vi "PicoReadPicoSingleBuffers.vi"(1 "enabled array":i16[](array[numeric]), 2 "Buffer and Transfer Settings":T3={"startIndex"=0, "Samples"=1000000, "Down Sample Ratio"=1, "Down-Sample Mode"=2147483648} {"Down-Sample Mode" items=["None"=2147483648, "Aggregate"=1, "Decimate"=2, "Average"=4]; "Down Sample Ratio" step=1; "Samples" format="%_6p"}, 3 "Variant":string, 5 "Data Pointers":T2, 9 "Buffer Number":i32=1, 11 "error in (no error)":errorcluster) -> (6 "MaxBuffers (Max or non-aggregated)":T1, 8 "Min Buffers":T1, 15 "error out":errorcluster)   [LabVIEW 2010]
doc: "Read data from a single Picodata buffer."
uses:
  PicoBuffers.ctl
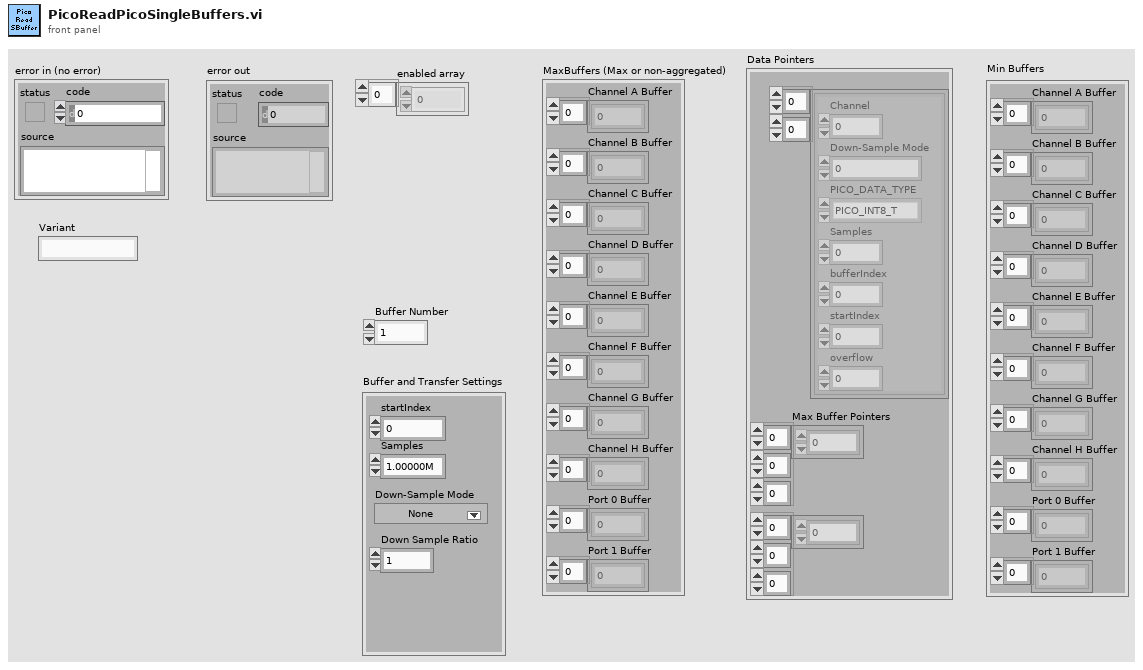
[diagram p1: front panel]
types:
  T1 = cluster{"Channel A Buffer":i16[], "Channel B Buffer":i16[], "Channel C Buffer":i16[], "Channel D Buffer":i16[], "Channel E Buffer":i16[], "Channel F Buffer":i16[], "Channel G Buffer":i16[], "Channel H Buffer":i16[], "Port 0 Buffer":i16[], "Port 1 Buffer":i16[]}
  T2 = typedef "PicoBuffers.ctl" = cluster{"Max Buffer Pointers":u64[][][], "Min Buffer Pointers":u64[][][], "StreamingDataInfo":cluster{"Channel":u32, "Down-Sample Mode":u32, "PICO_DATA_TYPE":enum32{"PICO_INT8_T", "PICO_INT16_T", "PICO_INT32_T", "PICO_UINT32_T", "PICO_INT64_T", ""}, "Samples":i32, "bufferIndex":u64, "startIndex":i32, "overflow":i16}[][]}
  T3 = cluster{"startIndex":u64, "Samples":u64, "Down Sample Ratio":u64, "Down-Sample Mode":u32}
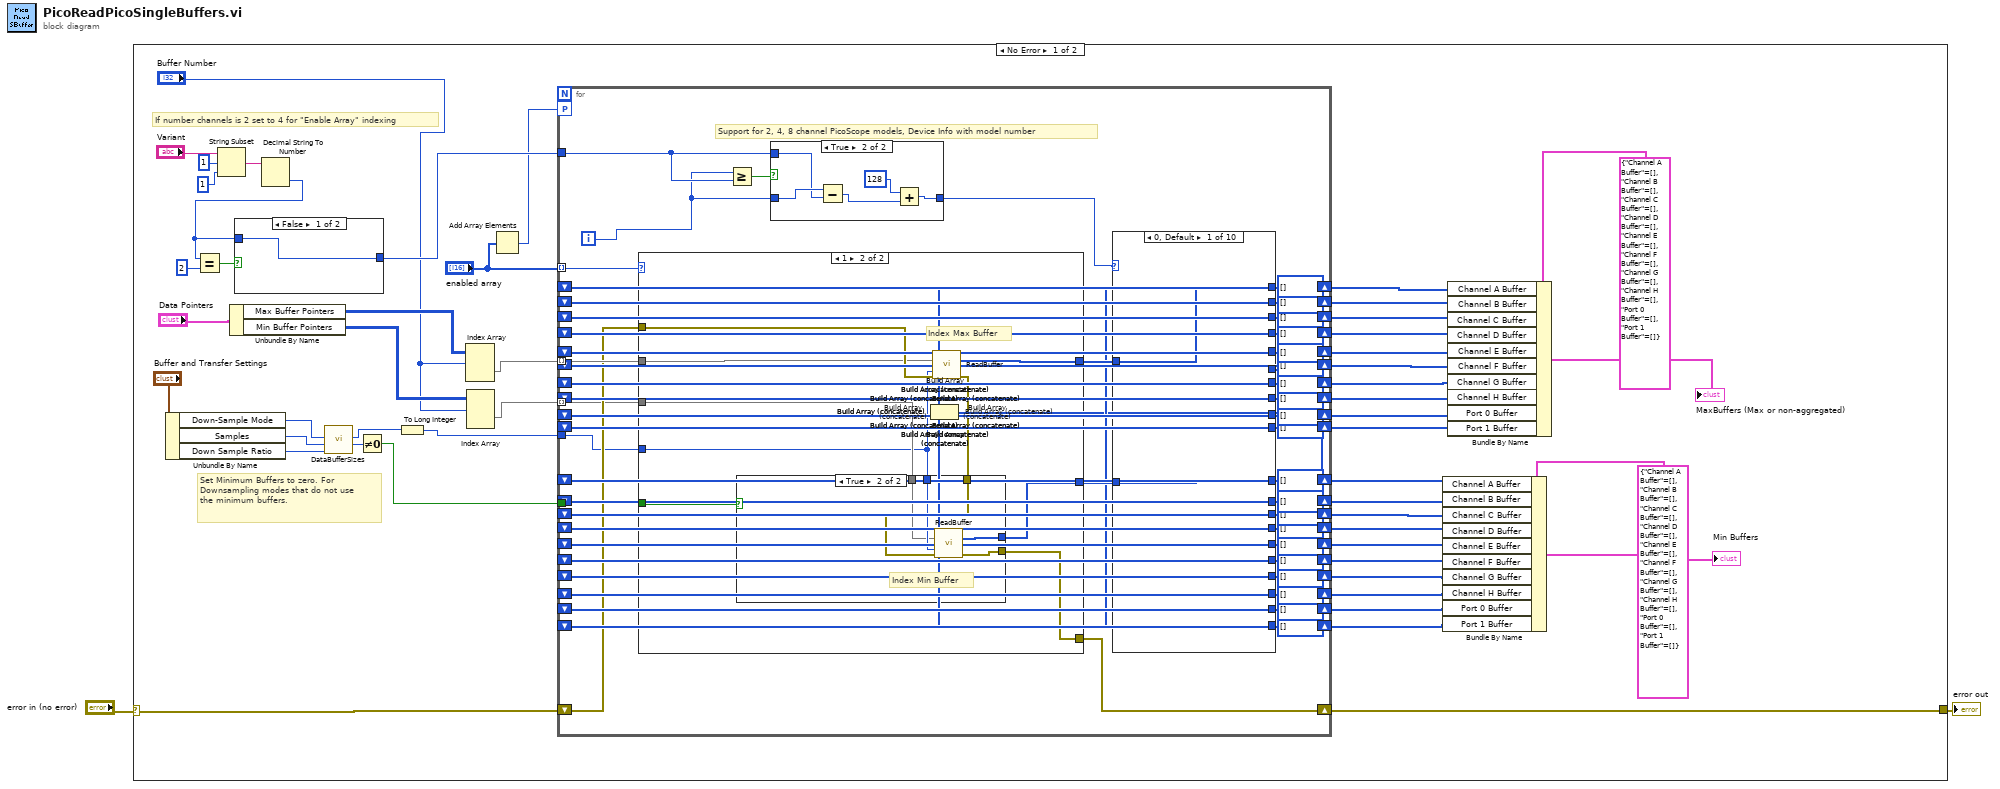
[diagram p0: block diagram]
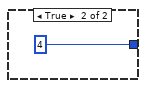
[diagram p14: hidden frame]
diagram:
  n1 = case shown="No Error" "error in (no error)" {
    selector: "error in (no error)" -> [w70 w190]
    tunnel: [w72 w190] -> w1
    frame No Error {
      # "If number channels is 2 set to 4 for \"Enable Array\" indexing"
      # "Set Minimum Buffers to zero. For Downsampling modes that do not use the minimum buffers."
      n2 = Unbundle By Name("Buffer and Transfer Settings") -> ("Down-Sample Mode"=w68:u32, "Samples"=w67:u64, "Down Sample Ratio"=w69:u64)
      n3 = String Subset(string="Variant", offset (0)=1, length (rest)=1 ("length (rest)")) -> (substring=w58:string)
      n4 = Unbundle By Name("Data Pointers") -> ("Max Buffer Pointers"=w29:u64[][][], "Min Buffer Pointers"=w28:u64[][][])
      n5 = Decimal String To Number(string=w58) -> (number=w55:i32)  [unwired: 2 in, 1 out]
      n6 = Equal?(x=w55, y=2 ("Number of channels")) -> (x = y?=w61:bool)
      n7 = case shown="False" w61 {
        tunnel: [w188 4 ("Number of channels")] -> w59
        tunnel: w55 -> [w188 _]
        frame False {
        }
        frame True {
        }
      }
      n8 = call "DataBufferSizes.vi"("Down Sample Ratio"=w69, "Number of Samples"=w67, "Down-Sample Mode"=w68) -> ("min Buffer Size"=w65:i32, "Max Buffer Size"=w63:i32)  [unwired: 7 in]
      n9 = Not Equal To 0?(x=w65) -> (x != 0?=w66:bool)
      n10 = To Long Integer(number=w63) -> (32bit integer=w64:i32)
      n11 = Index Array(array=w29, index (dim 0)="Buffer Number") -> (element=w27:u64[][])  [unwired: 2 in]
      n12 = Index Array(array=w28, index (dim 0)="Buffer Number") -> (element=w26:u64[][])  [unwired: 2 in]
      n13 = Add Array Elements(numeric array="enabled array") -> (sum=w23:i16)
      n14 = for {
        tunnel: "enabled array" -> [w144] mode=indexing
        tunnel: w27 -> [w145] mode=indexing
        shift-right: [w143] -> w72
        shift-left: w70 -> [w142]
        tunnel: w64 -> [w128]
        tunnel: w66 -> [w127]
        tunnel: w26 -> [w117] mode=indexing
        tunnel: w59 -> [w114]
        workers-P: w23 -> [_]
        shift-right: [w111] -> w53
        shift-left: i16[] [] ("Output Array") -> [w112]
        shift-right: [w109] -> w52
        shift-left: i16[] [] ("Output Array") -> [w110]
        shift-right: [w107] -> w51
        shift-left: i16[] [] ("Output Array") -> [w108]
        shift-right: [w105] -> w50
        shift-left: i16[] [] ("Output Array") -> [w106]
        shift-right: [w103] -> w49
        shift-left: i16[] [] ("Output Array") -> [w104]
        shift-right: [w101] -> w48
        shift-left: i16[] [] ("Output Array") -> [w102]
        shift-right: [w99] -> w42
        shift-left: i16[] [] ("Output Array") -> [w100]
        shift-right: [w97] -> w47
        shift-left: i16[] [] ("Output Array") -> [w98]
        shift-right: [w95] -> w46
        shift-left: i16[] [] ("Output Array") -> [w96]
        shift-right: [w93] -> w45
        shift-left: i16[] [] ("Output Array") -> [w94]
        shift-right: [w91] -> w44
        shift-left: i16[] [] ("Output Array") -> [w92]
        shift-right: [w89] -> w43
        shift-left: i16[] [] ("Output Array") -> [w90]
        shift-right: [w87] -> w39
        shift-left: i16[] [] ("Output Array") -> [w88]
        shift-right: [w85] -> w38
        shift-left: i16[] [] ("Output Array") -> [w86]
        shift-right: [w83] -> w37
        shift-left: i16[] [] ("Output Array") -> [w84]
        shift-right: [w81] -> w36
        shift-left: i16[] [] ("Output Array") -> [w82]
        shift-right: [w79] -> w35
        shift-left: i16[] [] ("Output Array") -> [w80]
        shift-right: [w77] -> w34
        shift-left: i16[] [] ("Output Array") -> [w78]
        shift-right: [w75] -> w33
        shift-left: i16[] [] ("Output Array") -> [w76]
        shift-right: [w73] -> w32
        shift-left: i16[] [] ("Output Array") -> [w74]
        i -> [w113]
        # "Support for 2, 4, 8 channel PicoScope models, Device Info with model number"
        n15 = case shown="1" w144 {
          tunnel: w145 -> [_ w175]
          tunnel: [_ w181] -> w141
          tunnel: [_ w180] -> w140
          tunnel: w142 -> [w172 w179]
          tunnel: [w172 w177] -> w143
          tunnel: w128 -> [_ w173]
          tunnel: w127 -> [_ w176]
          tunnel: w117 -> [_ w174]
          frame 0, Default {
          }
          frame 1 {
            # "Index Max Buffer"
            n16 = call "ReadBuffer.vi"("Pointer and BufferSize"=w175, "Buffer size"=w173, "error in (no error)"=w179) -> ("Output Array"=w181:i16[], "error out"=w178:errorcluster)  [unwired: 11 in]
            n17 = case shown="True" w176 {
              tunnel: [_ w187] -> w180
              tunnel: w178 -> [w182 w186]
              tunnel: [w182 w185] -> w177
              tunnel: w173 -> [_ w184]
              tunnel: w174 -> [_ w183]
              frame False {
              }
              frame True {
                # "Index Min Buffer"
                n18 = call "ReadBuffer.vi"("Pointer and BufferSize"=w183, "Buffer size"=w184, "error in (no error)"=w186) -> ("Output Array"=w187:i16[], "error out"=w185:errorcluster)  [unwired: 11 in]
              }
            }
          }
        }
        n19 = Greater Or Equal?(x=w113, y=w114) -> (x >= y?=w116:bool)
        n20 = case shown="True" w116 {
          tunnel: w113 -> [w146 w148]
          tunnel: [w146 w150] -> w115
          tunnel: w114 -> [_ w147]
          frame False {
          }
          frame True {
            n21 = Subtract(x=w148, y=w147) -> (x-y=w149:i32)
            n22 = Add(x=128, y=w149) -> (x+y=w150:i32)
          }
        }
        n23 = case shown="0, Default" w115 {
          tunnel: w141 -> [w153 w155 w157 w159 w161 w163 w165 w167 w169 w171]
          tunnel: [w153 _ _ _ _ _ _ _ _ _] -> w126
          tunnel: [_ w155 _ _ _ _ _ _ _ _] -> w133
          tunnel: [_ _ w157 _ _ _ _ _ _ _] -> w132
          tunnel: [_ _ _ w159 _ _ _ _ _ _] -> w131
          tunnel: [_ _ _ _ w161 _ _ _ _ _] -> w130
          tunnel: [_ _ _ _ _ w163 _ _ _ _] -> w129
          tunnel: w140 -> [w152 w154 w156 w158 w160 w162 w164 w166 w168 w170]
          tunnel: [w152 _ _ _ _ _ _ _ _ _] -> w139
          tunnel: [_ w154 _ _ _ _ _ _ _ _] -> w138
          tunnel: [_ _ w156 _ _ _ _ _ _ _] -> w137
          tunnel: [_ _ _ w158 _ _ _ _ _ _] -> w136
          tunnel: [_ _ _ _ w160 _ _ _ _ _] -> w135
          tunnel: [_ _ _ _ _ w162 _ _ _ _] -> w134
          tunnel: [_ _ _ _ _ _ w165 _ _ _] -> w125
          tunnel: [_ _ _ _ _ _ w164 _ _ _] -> w124
          tunnel: [_ _ _ _ _ _ _ w167 _ _] -> w123
          tunnel: [_ _ _ _ _ _ _ w166 _ _] -> w122
          tunnel: [_ _ _ _ _ _ _ _ w169 _] -> w121
          tunnel: [_ _ _ _ _ _ _ _ w168 _] -> w120
          tunnel: [_ _ _ _ _ _ _ _ _ w171] -> w119
          tunnel: [_ _ _ _ _ _ _ _ _ w170] -> w118
          frame 0, Default {
          }
          frame 1 {
          }
          frame 2 {
          }
          frame 3 {
          }
          frame 4 {
          }
          frame 5 {
          }
          frame 6 {
          }
          frame 7 {
          }
          frame 128 {
          }
          frame 129 {
          }
        }
        n24 = Build Array (concatenate)(w74, w118) -> (w73:i16[])
        n25 = Build Array (concatenate)(w76, w119) -> (w75:i16[])
        n26 = Build Array (concatenate)(w78, w120) -> (w77:i16[])
        n27 = Build Array (concatenate)(w80, w121) -> (w79:i16[])
        n28 = Build Array (concatenate)(w82, w122) -> (w81:i16[])
        n29 = Build Array (concatenate)(w84, w123) -> (w83:i16[])
        n30 = Build Array (concatenate)(w86, w124) -> (w85:i16[])
        n31 = Build Array (concatenate)(w88, w125) -> (w87:i16[])
        n32 = Build Array (concatenate)(w90, w129) -> (w89:i16[])
        n33 = Build Array (concatenate)(w92, w130) -> (w91:i16[])
        n34 = Build Array (concatenate)(w94, w131) -> (w93:i16[])
        n35 = Build Array (concatenate)(w96, w132) -> (w95:i16[])
        n36 = Build Array (concatenate)(w98, w133) -> (w97:i16[])
        n37 = Build Array (concatenate)(w100, w126) -> (w99:i16[])
        n38 = Build Array (concatenate)(w102, w134) -> (w101:i16[])
        n39 = Build Array (concatenate)(w104, w135) -> (w103:i16[])
        n40 = Build Array (concatenate)(w106, w136) -> (w105:i16[])
        n41 = Build Array (concatenate)(w108, w137) -> (w107:i16[])
        n42 = Build Array (concatenate)(w110, w138) -> (w109:i16[])
        n43 = Build Array (concatenate)(w112, w139) -> (w111:i16[])
      }
      n44 = Bundle By Name(cluster=T1 {"Channel A Buffer"=[], "Channel B Buffer"=[], "Channel C Buffer"=[], "Channel D Buffer"=[], "Channel E Buffer"=[], "Channel F Buffer"=[], "Channel G Buffer"=[], "Channel H Buffer"=[], "Port 0 Buffer"=[], "Port 1 Buffer"=[]} ("input cluster"), "Channel A Buffer"=w53, "Channel B Buffer"=w52, "Channel C Buffer"=w51, "Channel D Buffer"=w50, "Channel E Buffer"=w49, "Channel F Buffer"=w48, "Channel G Buffer"=w38, "Channel H Buffer"=w36, "Port 0 Buffer"=w34, "Port 1 Buffer"=w32) -> (→"Min Buffers":T1)
      n45 = Bundle By Name(cluster=T1 {"Channel A Buffer"=[], "Channel B Buffer"=[], "Channel C Buffer"=[], "Channel D Buffer"=[], "Channel E Buffer"=[], "Channel F Buffer"=[], "Channel G Buffer"=[], "Channel H Buffer"=[], "Port 0 Buffer"=[], "Port 1 Buffer"=[]} ("input cluster"), "Channel A Buffer"=w42, "Channel B Buffer"=w47, "Channel C Buffer"=w46, "Channel D Buffer"=w45, "Channel E Buffer"=w44, "Channel F Buffer"=w43, "Channel G Buffer"=w39, "Channel H Buffer"=w37, "Port 0 Buffer"=w35, "Port 1 Buffer"=w33) -> (→"MaxBuffers (Max or non-aggregated)":T1)
    }
    frame Error {
    }
  }
  "error out" <- w1
